vi "AddMa.vi"(8 "Dest 3":dbl[](array[numeric]), 9 "Toa Do":dbl[](array[numeric]), 10 "MaBegin":string, 11 "String IN":string) -> (3 "String OUT":string)   [LabVIEW 2017]
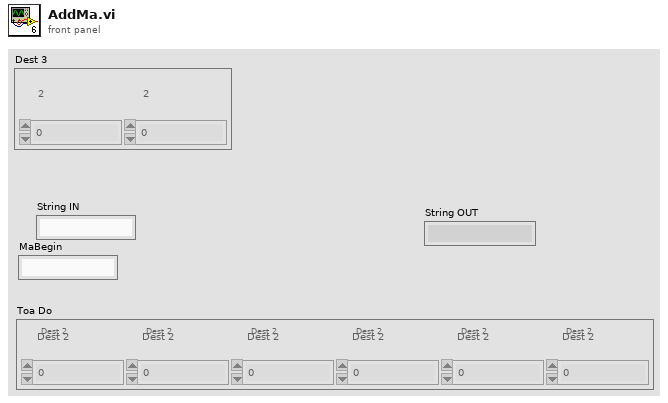
[diagram p1: front panel]
types:
  T1 = cluster{"Toa Do[0]":dbl, "Toa Do[1]":dbl, "Toa Do[2]":dbl, "Toa Do[3]":dbl, "Toa Do[4]":dbl, "Toa Do[5]":dbl, "Toa Do[6]":dbl, "Toa Do[7]":dbl, "Toa Do[8]":dbl, "Toa Do[9]":dbl, "Toa Do[10]":dbl, "Toa Do[11]":dbl}
  T2 = cluster{"Dest 3[0]":dbl, "Dest 3[1]":dbl, "Dest 3[2]":dbl, "Dest 3[3]":dbl, "Dest 3[4]":dbl, "Dest 3[5]":dbl, "Dest 3[6]":dbl, "Dest 3[7]":dbl, "Dest 3[8]":dbl, "Dest 3[9]":dbl, "Dest 3[10]":dbl, "Dest 3[11]":dbl}
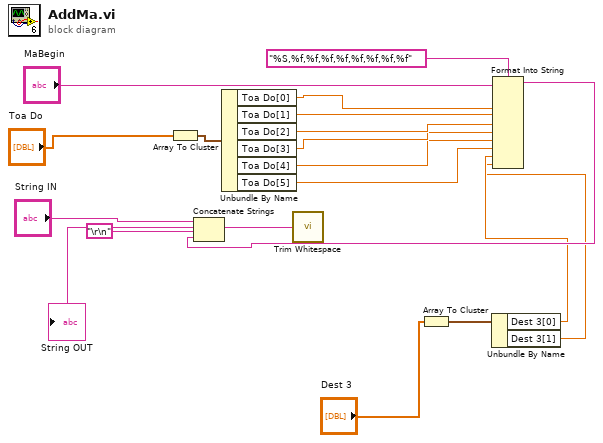
[diagram p0: block diagram]
diagram:
  n1 = Array To Cluster(array="Toa Do") -> (cluster=w11:T1)
  n2 = Unbundle By Name(w11) -> ("Toa Do[0]"=w10:dbl, "Toa Do[1]"=w9:dbl, "Toa Do[2]"=w8:dbl, "Toa Do[3]"=w7:dbl, "Toa Do[4]"=w6:dbl, "Toa Do[5]"=w5:dbl)
  n3 = Array To Cluster(array="Dest 3") -> (cluster=w3:T2)
  n4 = Unbundle By Name(w3) -> ("Dest 3[0]"=w2:dbl, "Dest 3[1]"=w1:dbl)
  n5 = Format Into String(format string="%S,%f,%f,%f,%f,%f,%f,%f,%f", "MaBegin", w10, w9, w8, w7, w6, w5, w2, w1) -> (resulting string=w15:string)  [unwired: 2 in, 1 out]
  n6 = Concatenate Strings("String IN", "\r\n", w15) -> (w19:string)
  n7 = call <vilib>:"Trim Whitespace.vi"("string"=w19) -> ("trimmed string"=→"String OUT":string)  [unwired: 1 in]
